vi "Path_HDH VIPM Folder.vi"() -> (2 "Success?":bool, 3 "HDH\\VIPM path":path)   [LabVIEW 2019, in "Project.Dependencies Finder.lvlib" / "Dependency Source_VIPM.lvclass"]
uses:
  Dependency Source_VIPM.lvclass
  <vilib>/Utility/sysdir.llb/System Directory Type.ctl
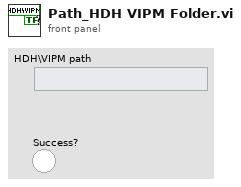
[diagram p1: front panel]
types:
  T1 = typedef "System Directory Type.ctl" = i32
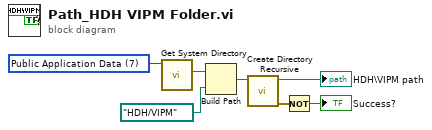
[diagram p0: block diagram]
diagram:
  w7 = T1 7 items=["User Home"=0, "User Desktop"=1, "User Documents"=2, "User Application Data"=3, "User Preferences"=4, "User Temporary"=5, "Public Documents"=6, "Public Application Data"=7, "Public Preferences"=8, "Public Cache"=13, "System Core Libraries"=9, "System Installed Libraries"=10, "Application Files"=11, "Boot Volume Root"=12] ("system directory type")
  n1 = call <vilib>:"Get System Directory.vi"("system directory type"=w7) -> ("system directory"=w5:path)  [unwired: 10 in]
  n2 = Build Path(base path=w5, name or relative path=path "HDH/VIPM") -> (appended path=w4:path)
  n3 = call <vilib>:"Create Directory Recursive.vi"("directory"=w4) -> ("error out"=w2:errorcluster, "directory copy"=→"HDH\\VIPM path":path)  [unwired: 4 in, 1 out]
  n4 = Not(x=w2) -> (.not. x?=→"Success?":bool)
